vi "Remove Result Sections.vi"(8 "Error in":errorcluster, 11 "Custom Device ref":T1 format="%.0x") -> (0 "Error out":errorcluster, 3 "Custom Device ref out":T1 format="%.0x")   [LabVIEW 2014, in "Waveform-Processing-Custom-Device System Explorer.lvlib"]
uses:
  Waveform-Processing-Custom-Device System Explorer.lvlib
  <vilib>/NI Veristand/Custom Device API/Custom Device Item Ref.ctl
  Shared/Constants.vi
  <vilib>/NI Veristand/Custom Device API/Custom Device API.lvlib
  Shared/Waveform-Processing-Custom-Device Shared.lvlib
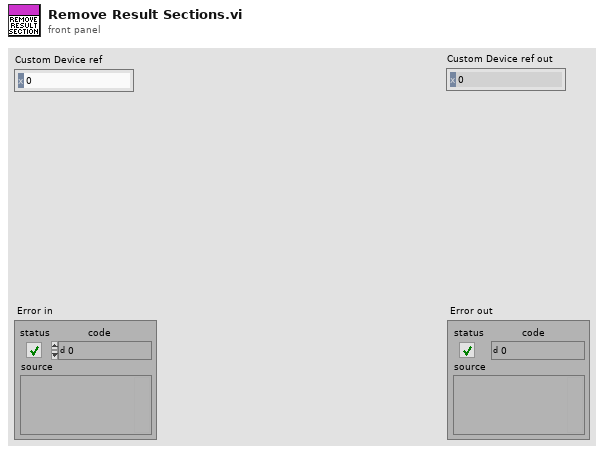
[diagram p1: front panel]
types:
  T1 = typedef "Custom Device API.lvlib/Custom Device Item Ref.ctl" = u64
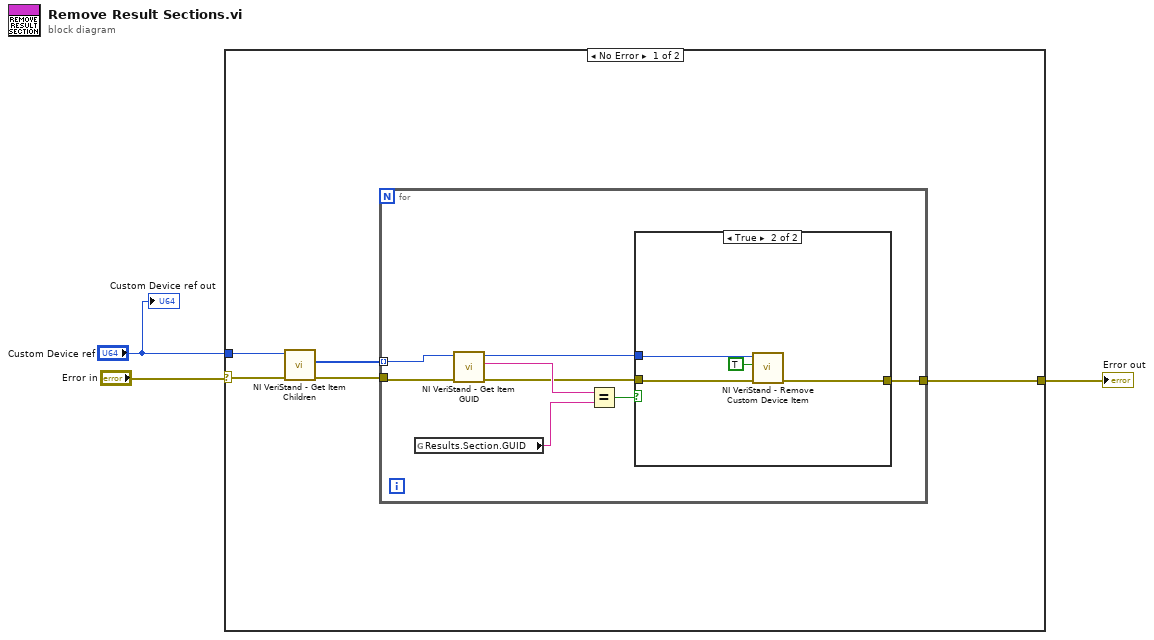
[diagram p0: block diagram]
diagram:
  n1 = case shown="No Error" "Error in" {
    selector: "Error in" -> [w8 w22]
    tunnel: "Custom Device ref" -> [w7 _]
    tunnel: [w4 w22] -> w2
    frame No Error {
      n2 = call <vilib>:"NI VeriStand - Get Item Children.vi"("error in (no error)"=w8, "Item Ref in"=w7) -> ("error out"=w6:errorcluster, "Child Refs"=w5:T1[])  [unwired: 6 in, 2 out]
      n3 = for {
        tunnel: w6 -> [w16]
        tunnel: w5 -> [w15] mode=indexing
        tunnel: [w9] -> w4
        n4 = global read "Constants.vi" "Results.Section.GUID"() -> (w13:string)
        n5 = call <vilib>:"NI VeriStand - Get Item GUID.vi"("error in (no error)"=w16, "Item Ref in"=w15) -> ("error out"=w11:errorcluster, "GUID"=w14:string, "Item Ref out"=w10:T1)  [unwired: 7 in]
        n6 = Equal?(x=w14, y=w13) -> (x = y?=w12:bool)
        n7 = case shown="True" w12 {
          tunnel: w11 -> [w17 w19]
          tunnel: w10 -> [_ w21]
          tunnel: [w17 w18] -> w9
          frame False {
          }
          frame True {
            n8 = call <vilib>:"NI VeriStand - Remove Custom Device Item.vi"("error in (no error)"=w19, "Force Delete (F)"=TRUE, "Item Ref in"=w21) -> ("error out"=w18:errorcluster)  [unwired: 7 in, 1 out]
          }
        }
      }
    }
    frame Error {
    }
  }
  "Error out" <- w2
  "Custom Device ref out" <- "Custom Device ref"
